vi "Set Tray Icon (string).vi"(0 "NotifyIcon in":refnum<class "NotifyIcon.lvclass">, 7 "Icon String":string, 11 "error in (no error)":errorcluster) -> (4 "NotifyIcon out":refnum<class "NotifyIcon.lvclass">, 15 "error out":errorcluster)   [LabVIEW 2016, in "NotifyIcon.lvclass"]
doc: "This VI is used to set the icon that is associated with the context menu and shown in the notification area.\nThe VI translates the input <b>Icon String</b> into a memory stream and then uses this as the source of the icon. <b>Icon String</b> is expected to be a binary representation of an ICO file!\n\nThis VI is usefull because the icon source can then be included in the VI code as a string constant.\n\n\nStinus Olsen\nCIM Industrial Systems A/S\n22. Feb. 2011 15:06\nmailto: seo@cim.as"
uses:
  NotifyIcon.lvclass
  System.Drawing
panel:
  # "This VI belongs to the NotifyIcon Toolset. \nA toolset that makes it easy to create, control and manipulate a notification icon in the notification area of the Windows taskbar.\nThe toolset requires Microsoft .NET framework 2.0\n\n\nNOTICE -- YOU MUST LEAVE THIS NOTICE IN PLACE.  PER THE TERMS OF THE LICENSE BELOW, YOU MAY SUBLICENSE THIS SOFTWARE \nIN ANY WAY THAT DOES NOT CONFLICT WITH THIS LICENSE.\n\n### BSD License (http://www.opensource.org/licenses/bsd-license.php) Begin ###\n \nCopyright (c) 2011, Stinus Olsen <seo@cim.as>\n\nAll rights reserved.\n\nRedistribution and use in source and binary forms, with or without modification, are permitted provided that the following conditions are met:\n\n    * Redistributions of source code must retain the above copyright notice, this list of conditions and the following disclaimer.\n    * Redistributions in binary form must reproduce the above copyright notice, this list of conditions and the following disclaimer in the \n       documentation and/or other materials provided with the distribution.\n    * Neither the name of CIM Industrial Systems nor the names of its contributors may be used to endorse or promote products derived \n       from this software without specific prior written permission.\n\nTHIS SOFTWARE IS PROVIDED BY THE COPYRIGHT HOLDERS AND CONTRIBUTORS \"AS IS\" AND ANY EXPRESS OR IMPLIED WARRANTIES, \nINCLUDING, BUT NOT LIMITED TO, THE IMPLIED WARRANTIES OF MERCHANTABILITY AND FITNESS FOR A PARTICULAR PURPOSE ARE \nDISCLAIMED. IN NO EVENT SHALL THE COPYRIGHT OWNER OR CONTRIBUTORS BE LIABLE FOR ANY DIRECT, INDIRECT, INCIDENTAL,\n SPECIAL, EXEMPLARY, OR CONSEQUENTIAL DAMAGES (INCLUDING, BUT NOT LIMITED TO, PROCUREMENT OF SUBSTITUTE GOODS OR \nSERVICES; LOSS OF USE, DATA, OR PROFITS; OR BUSINESS INTERRUPTION) HOWEVER CAUSED AND ON ANY THEORY OF LIABILITY, \nWHETHER IN CONTRACT, STRICT LIABILITY, OR TORT (INCLUDING NEGLIGENCE OR OTHERWISE) ARISING IN ANY WAY OUT OF THE USE \nOF THIS SOFTWARE, EVEN IF ADVISED OF THE POSSIBILITY OF SUCH DAMAGE.\n\n### BSD License End ###"
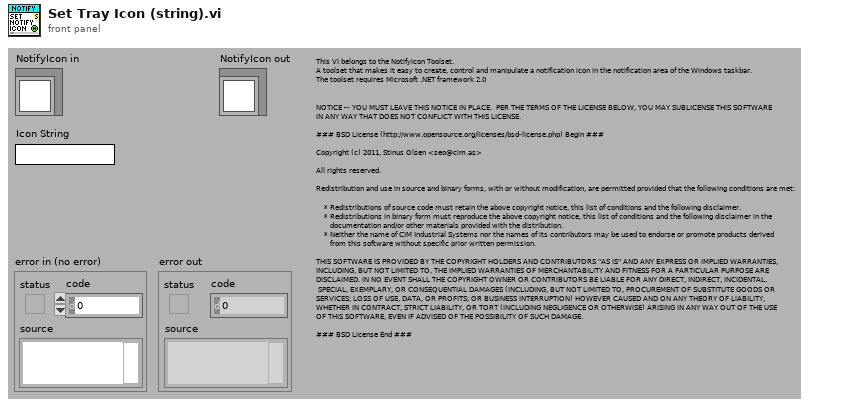
[diagram p1: front panel]
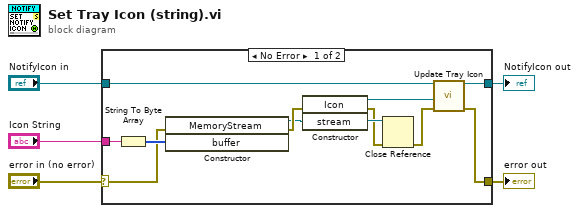
[diagram p0: block diagram]
diagram:
  n1 = case shown="No Error" "error in (no error)" {
    selector: "error in (no error)" -> [w9 w18]
    tunnel: [w14 w18] -> w4
    tunnel: [w15 w17] -> w2
    tunnel: "NotifyIcon in" -> [w16 w17]
    tunnel: "Icon String" -> [w12 _]
    frame No Error {
      n2 = String To Byte Array(string=w12) -> (unsigned byte array=w11:u8[])
      n3 = constructor class="MemoryStream"(error in=w9, "buffer"=w11) -> (reference out=w8:refnum<k24>, error out=w10:errorcluster)  [unwired: 2 in, 2 out]
      n4 = constructor class="Icon"(error in=w10, "stream"=w8) -> (reference out=w13:refnum<k24>, error out=w7:errorcluster)  [unwired: 2 in, 2 out]
      n5 = Close Reference(reference=w8, error in (no error)=w7) -> (error out=w6:errorcluster)
      n6 = call "Update Tray Icon.vi"("NotifyIcon in"=w16, "Icon Reference"=w13, "error in (no error)"=w6) -> ("NotifyIcon out"=w15:refnum<class "NotifyIcon.lvclass">, "error out"=w14:errorcluster)  [unwired: 1 in, 10 out]
    }
    frame Error {
    }
  }
  "error out" <- w4
  "NotifyIcon out" <- w2
